vi "Placas_Foco.vi"() -> ()   [LabVIEW 2021]
uses:
  <vilib>/userdefined/High Color/IMAQdx.ctl
  <vilib>/Instr/_visa.llb/VISA Configure Serial Port (Instr).vi
  <vilib>/vision/driver/NI_Vision_Acquisition_Software.lvlib
  <vilib>/vision/NI_Vision_Development_Module.lvlib
panel:
  in  "VISA resource name":refnum<visa-resource-name>
  out "String":string
  out "Matches[0].Position.y":sgl
  out "Matches[0].Position.x":sgl
  in  "Reconocer":bool
  in  "Stop":bool
  in  "Camara":T1
  out "Imagen":T2(plugin-control)
  out "Muestra":T2(plugin-control)
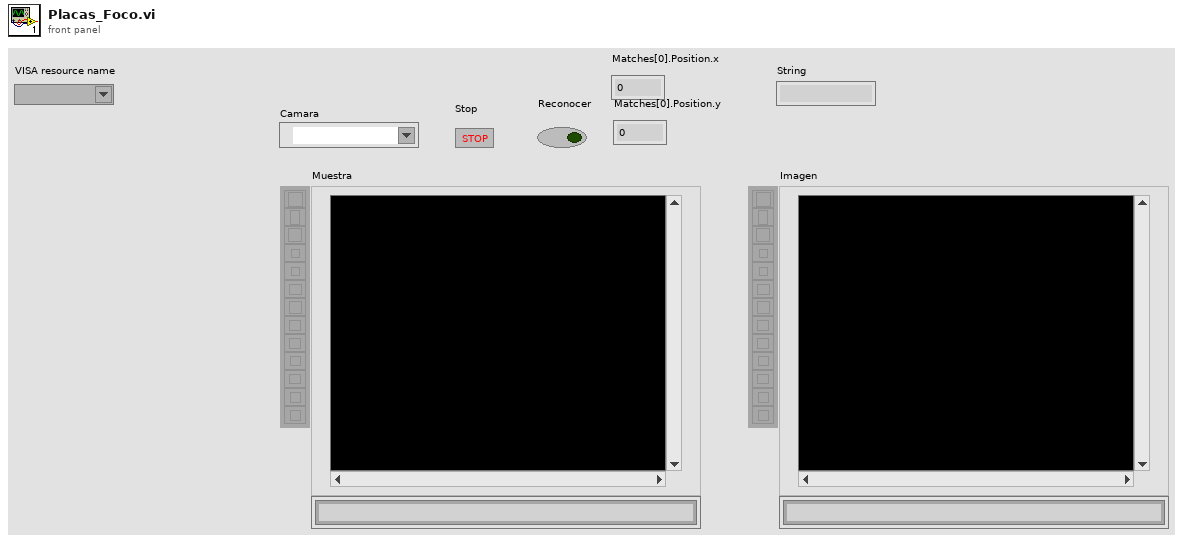
[diagram p1: front panel]
types:
  T1 = typedef "IMAQdx.ctl" = refnum<k21>
  T2 = typedef "IMAQ Image.ctl" = refnum<image>
  T3 = typedef "Image Type" = u32
  T4 = cluster{"Match Mode":u16, "Number of Matches Requested":i32, "Minimum Match Score":sgl, "SubPixel Accuracy":bool, "Rotation Angle Ranges":cluster{"Start":sgl, "End":sgl}[], "Show Search Area":bool, "Show Result":bool}
  T5 = cluster{"Position":cluster{"x":sgl, "y":sgl}, "Angle":sgl, "Scale":sgl, "Score":sgl, "Bounding Box":cluster{"x":sgl, "y":sgl}[]}[]
  T6 = cluster{"Matches[0]":cluster{"Position":cluster{"x":sgl, "y":sgl}, "Angle":sgl, "Scale":sgl, "Score":sgl, "Bounding Box":cluster{"x":sgl, "y":sgl}[]}, "Matches[1]":cluster{"Position":cluster{"x":sgl, "y":sgl}, "Angle":sgl, "Scale":sgl, "Score":sgl, "Bounding Box":cluster{"x":sgl, "y":sgl}[]}, "Matches[2]":cluster{"Position":cluster{"x":sgl, "y":sgl}, "Angle":sgl, "Scale":sgl, "Score":sgl, "Bounding Box":cluster{"x":sgl, "y":sgl}[]}, "Matches[3]":cluster{"Position":cluster{"x":sgl, "y":sgl}, "Angle":sgl, "Scale":sgl, "Score":sgl, "Bounding Box":cluster{"x":sgl, "y":sgl}[]}, "Matches[4]":cluster{"Position":cluster{"x":sgl, "y":sgl}, "Angle":sgl, "Scale":sgl, "Score":sgl, "Bounding Box":cluster{"x":sgl, "y":sgl}[]}, "Matches[5]":cluster{"Position":cluster{"x":sgl, "y":sgl}, "Angle":sgl, "Scale":sgl, "Score":sgl, "Bounding Box":cluster{"x":sgl, "y":sgl}[]}, "Matches[6]":cluster{"Position":cluster{"x":sgl, "y":sgl}, "Angle":sgl, "Scale":sgl, "Score":sgl, "Bounding Box":cluster{"x":sgl, "y":sgl}[]}, "Matches[7]":cluster{"Position":cluster{"x":sgl, "y":sgl}, "Angle":sgl, "Scale":sgl, "Score":sgl, "Bounding Box":cluster{"x":sgl, "y":sgl}[]}, "Matches[8]":cluster{"Position":cluster{"x":sgl, "y":sgl}, "Angle":sgl, "Scale":sgl, "Score":sgl, "Bounding Box":cluster{"x":sgl, "y":sgl}[]}}
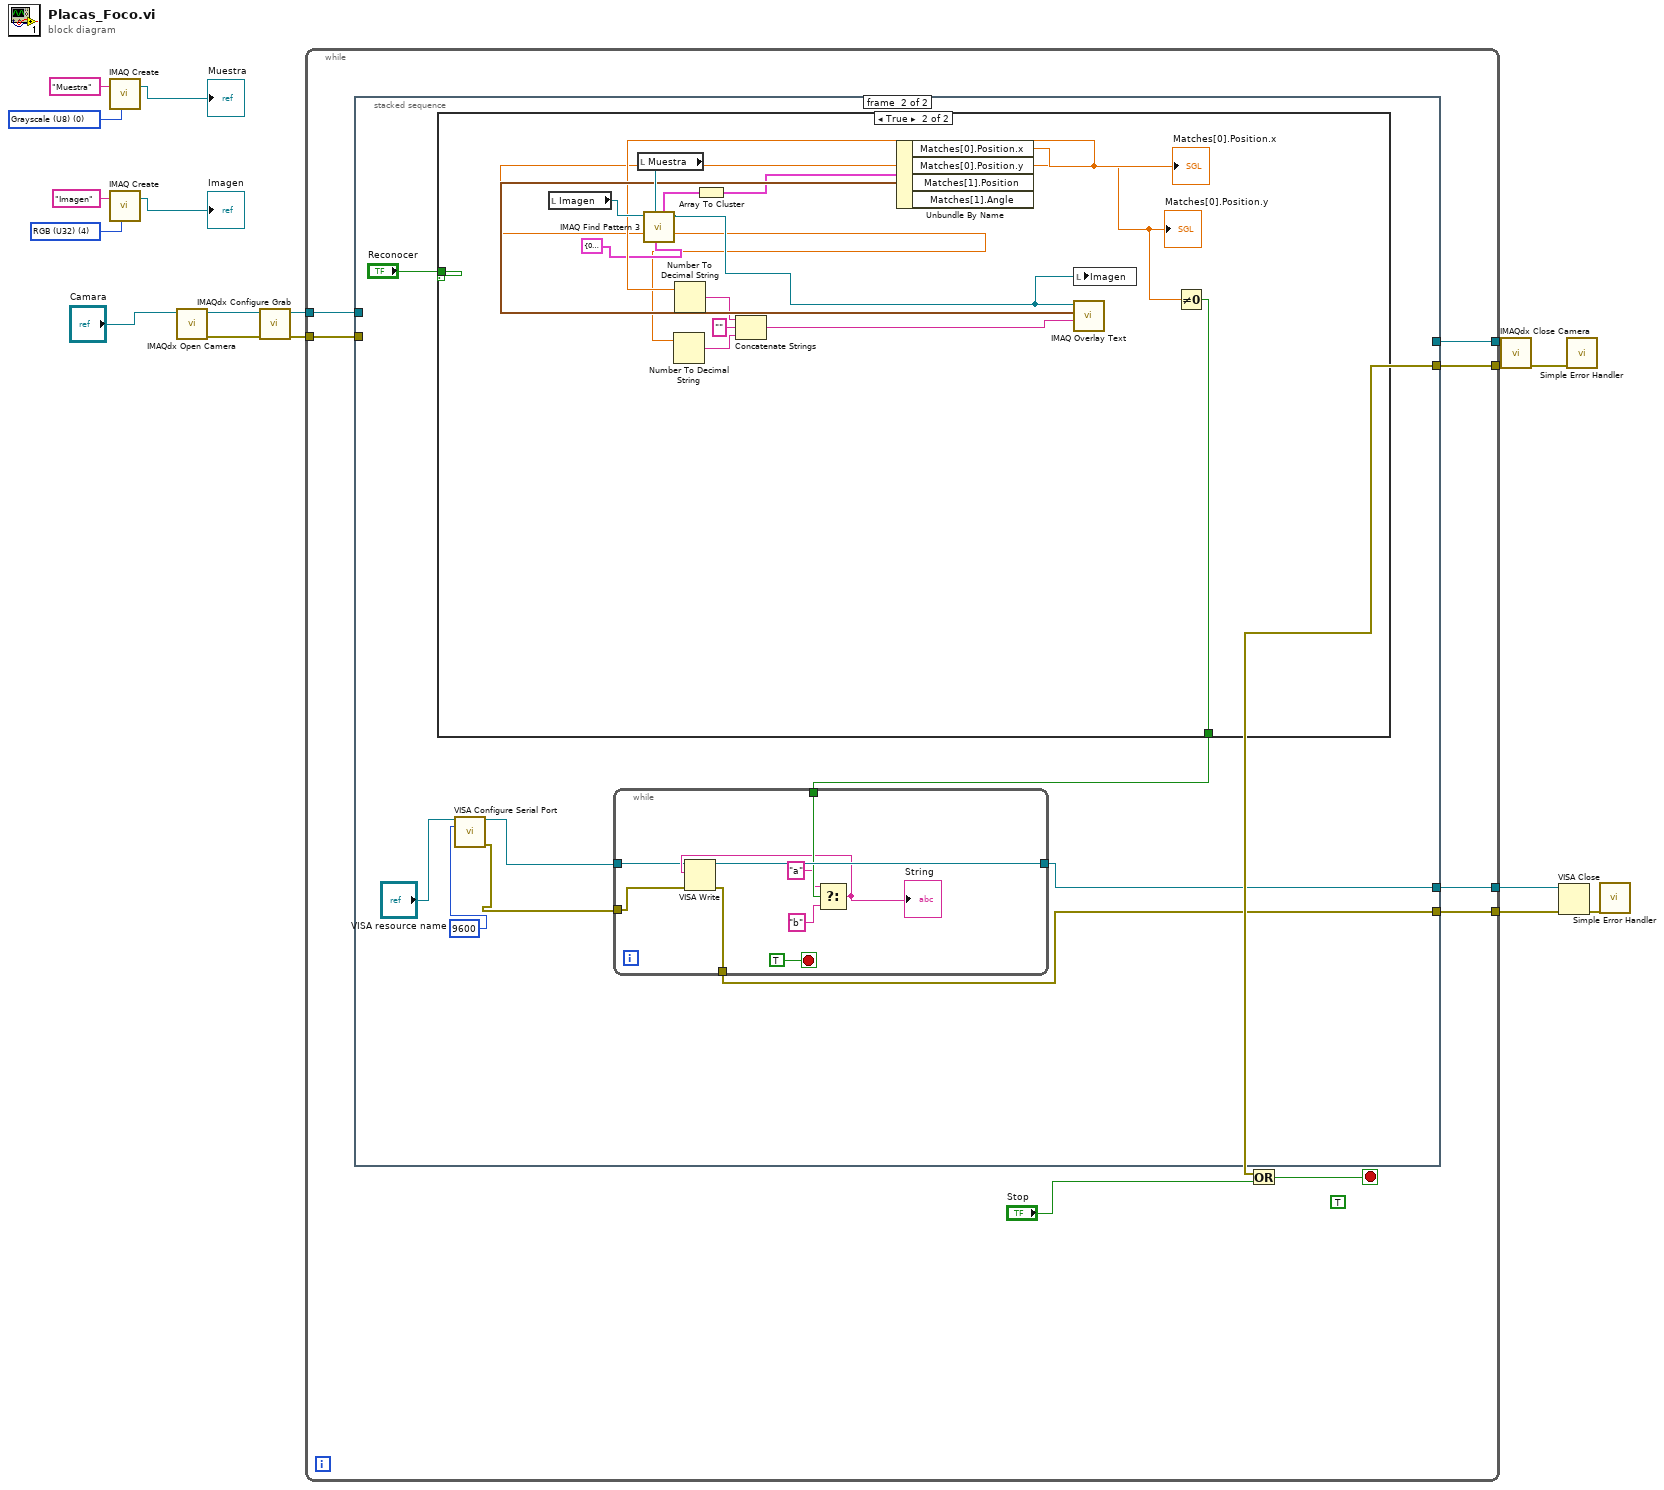
[diagram p0: block diagram]
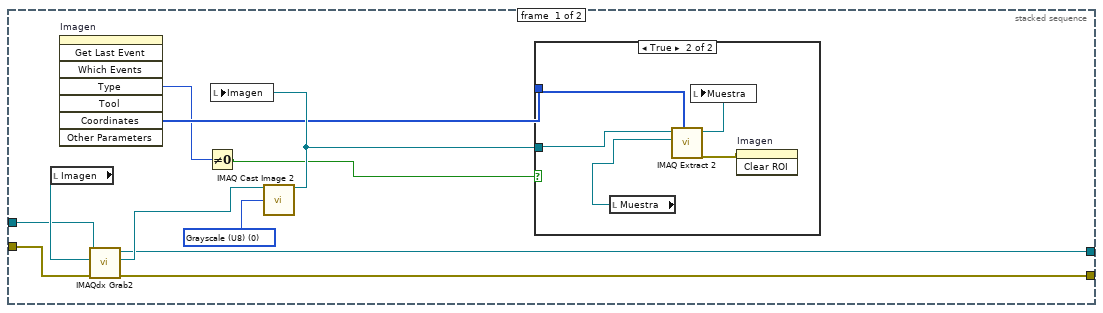
[diagram p2: hidden frame]
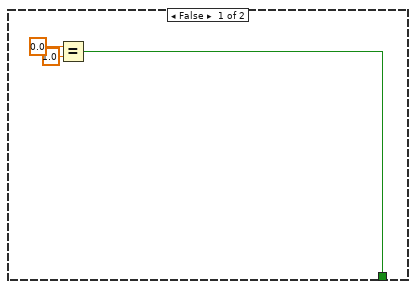
[diagram p4: hidden frame]
diagram:
  w13 = T3 4 items=["Grayscale (U8)", "Grayscale (I16)", "Grayscale (SGL)", "Complex (CSG)", "RGB (U32)", "HSL (U32)", "RGB (U64)", "Grayscale (U16)"] ("Image Type")
  w16 = T3 0 items=["Grayscale (U8)", "Grayscale (I16)", "Grayscale (SGL)", "Complex (CSG)", "RGB (U32)", "HSL (U32)", "RGB (U64)", "Grayscale (U16)"] ("Image Type")
  n1 = call "IMAQ Create"("Image Name"="Muestra", "Image Type"=w16) -> ("New Image"=→"Muestra":T2)  [unwired: 3 in, 1 out]
  n2 = call "IMAQ Create"("Image Name"="Imagen", "Image Type"=w13) -> ("New Image"=→"Imagen":T2)  [unwired: 3 in, 1 out]
  n3 = call <vilib>:"IMAQdx Open Camera.vi"("Session In"="Camara") -> ("error out"=w9:errorcluster, "Session Out"=w10:T1)  [unwired: 9 in]
  n4 = call <vilib>:"IMAQdx Configure Grab.vi"("error in"=w9, "Session In"=w10) -> ("error out"=w7:errorcluster, "Session Out"=w8:T1)  [unwired: 8 in]
  n5 = while {
    tunnel: w8 -> [w25]
    tunnel: w7 -> [w24]
    tunnel: [w23] -> w6
    tunnel: [w20] -> w5
    tunnel: [w19] -> w2
    tunnel: [w18] -> w1
    stop <- w21 stop-if-true
    (unwired) TRUE
    n6 = stacked-sequence {
      tunnel: w25 -> [w35 _]
      tunnel: w24 -> [w31 _]
      tunnel: [w27 _] -> w23
      tunnel: [w26 _] -> w20
      tunnel: [_ w47] -> w19
      tunnel: [_ w46] -> w18
      frame #0 {
        w33 = T3 0 items=["Grayscale (U8)", "Grayscale (I16)", "Grayscale (SGL)", "Complex (CSG)", "RGB (U32)", "HSL (U32)", "RGB (U64)", "Grayscale (U16)"] ("Image Type")
        n7 = local read "Imagen"() -> (w36:T2)
        n8 = invoke on="Imagen" class="ImageControl" method="Get Last Event"() -> ("Type"=w29:i32, "Coordinates"=w30:i32[])  [unwired: 8 in, 6 out]
        n9 = call <vilib>:"IMAQdx Grab2.vi"("error in"=w31, "Image In"=w36, "Session In"=w35) -> ("error out"=w26:errorcluster, "Image Out"=w34:T2, "Session Out"=w27:T1)  [unwired: 5 in, 1 out]
        n10 = Not Equal To 0?(x=w29) -> (x != 0?=w28:bool)
        n11 = call "IMAQ Cast Image 2"("Image Src"=w34, "Image Type"=w33) -> ("Image Dst Out"=w32:T2)  [unwired: 12 in, 1 out]
        n12 = local write "Imagen"(w32) -> ()
        n13 = case shown="True" w28 {
          tunnel: w32 -> [_ w41]
          tunnel: w30 -> [_ w38]
          frame False {
          }
          frame True {
            n14 = local read "Muestra"() -> (w40:T2)
            n15 = call "IMAQ Extract 2"("Optional Rectangle"=w38, "Image Dst"=w40, "Image Src"=w41) -> ("error out"=w37:errorcluster, "Image Dst Out"=w39:T2)  [unwired: 7 in]
            n16 = local write "Muestra"(w39) -> ()
            n17 = invoke on="Imagen" class="ImageControl" method="Clear ROI"(error in=w37) -> ()  [unwired: 2 in, 3 out]
          }
        }
      }
      frame #1 {
        n18 = case shown="True" "Reconocer" {
          tunnel: "Reconocer" -> [_ _]
          tunnel: [w59 w62] -> w48
          frame False {
            n19 = Equal?(x=0.0, y=1.0) -> (x = y?=w59:bool)
          }
          frame True {
            n20 = local read "Imagen"() -> (w74:T2)
            n21 = local read "Muestra"() -> (w75:T2)
            n22 = call "IMAQ Find Pattern 3"("Settings"=T4 {"Match Mode"=0, "Number of Matches Requested"=1, "Minimum Match Score"=800.0, "SubPixel Accuracy"=FALSE, "Rotation Angle Ranges"=[], "Show Search Area"=FALSE, "Show Result"=TRUE}, "Template"=w75, "Image"=w74) -> ("Image Out"=w73:T2, "Matches"=w66:T5)  [unwired: 3 in, 4 out]
            n23 = Array To Cluster(array=w66) -> (cluster=w67:T6)
            n24 = Unbundle By Name(w67) -> ("Matches[0].Position.x"=w69:sgl, "Matches[0].Position.y"=w63:sgl, "Matches[1].Position"=w72:cluster{"x":sgl, "y":sgl})  [unwired: 1 out]
            "Matches[0].Position.x" <- w69
            "Matches[0].Position.y" <- w63
            n25 = Number To Decimal String(number=w63) -> (decimal integer string=w70:string)  [unwired: 1 in]
            n26 = Number To Decimal String(number=w69) -> (decimal integer string=w68:string)  [unwired: 1 in]
            n27 = Concatenate Strings(w68, "" ("string"), w70) -> (w71:string)
            n28 = local write "Imagen"(w73) -> ()
            n29 = call "IMAQ Overlay Text"("String"=w71, "Origin"=w72, "Image"=w73) -> ()  [unwired: 7 in, 2 out]
            n30 = Not Equal To 0?(x=w63) -> (x != 0?=w62:bool)
          }
        }
        n31 = call-poly "VISA Configure Serial Port"("VISA resource name"="VISA resource name", "baud rate (9600)"=u32 9600) -> ("VISA resource name out"=w42:refnum<visa-resource-name>, "error out"=w43:errorcluster)  [unwired: 12 in]
        n32 = while {
          tunnel: [w58] -> w46
          tunnel: [w57] -> w47
          tunnel: w48 -> [w54]
          tunnel: w42 -> [w51]
          tunnel: w43 -> [w50]
          stop <- TRUE stop-if-true
          n33 = Select(t="a", s=w54, f="b") -> (s? t:f=w52:string)
          "String" <- w52
          n34 = VISA Write(VISA resource name=w51, write buffer=w52, error in (no error)=w50) -> (VISA resource name out=w58:refnum<visa-resource-name>, error out=w57:errorcluster)  [unwired: 1 out]
        }
      }
    }
    n35 = Or(x=w20, y="Stop") -> (x .or. y?=w21:bool)
  }
  n36 = call <vilib>:"IMAQdx Close Camera.vi"("error in"=w5, "Session In"=w6) -> ("error out"=w4:errorcluster)  [unwired: 9 in]
  n37 = VISA Close(VISA resource name=w1, error in (no error)=w2) -> (error out=w3:errorcluster)
  n38 = call <vilib>:"Simple Error Handler.vi"("error in (no error)"=w4) -> ()  [unwired: 4 in, 5 out]
  n39 = call <vilib>:"Simple Error Handler.vi"("error in (no error)"=w3) -> ()  [unwired: 4 in, 5 out]
